vi "extract Z segment with cursors.vi"(6 "sample rate":dbl, 8 "Zmag trajectory":waveform(dbl) caption="元素", 9 "cursor pos":dbl, 10 "data":waveform(dbl)[](array[waveform]), 11 "cursor length":dbl) -> (0 "Z":dbl[](array[numeric]), 4 "Z mag":dbl[](array[numeric]))   [LabVIEW 2017]
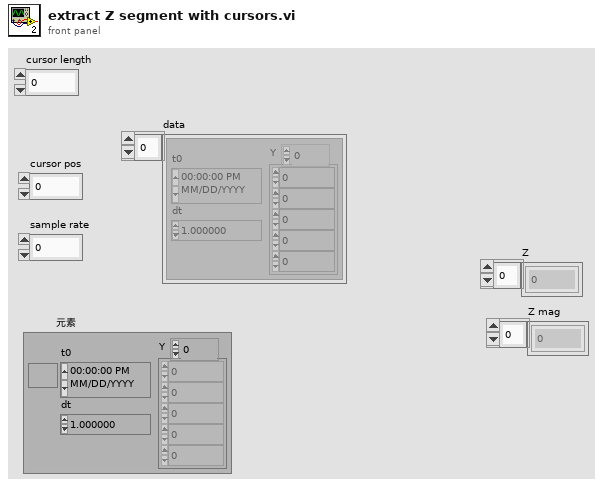
[diagram p1: front panel]
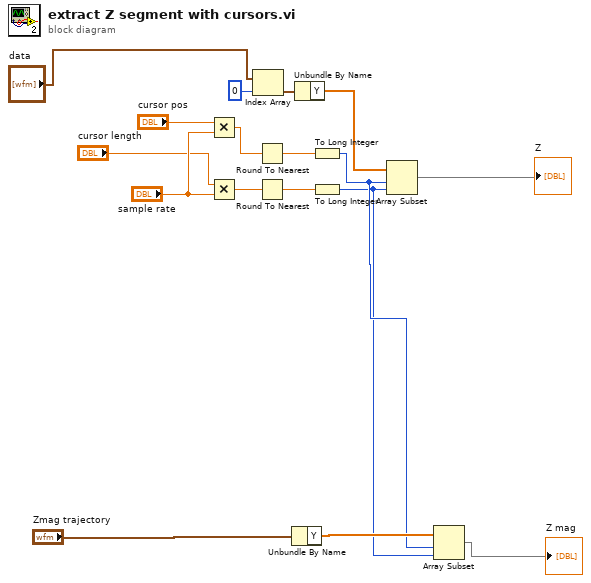
[diagram p0: block diagram]
diagram:
  n1 = Multiply(x="cursor pos", y="sample rate") -> (x*y=w11:dbl)
  n2 = Multiply(x="cursor length", y="sample rate") -> (x*y=w15:dbl)
  n3 = Index Array(array="data", index=0 ("索引")) -> (element=w9:waveform(dbl))
  n4 = Round To Nearest(number=w11) -> (nearest integer value=w12:dbl)
  n5 = Round To Nearest(number=w15) -> (nearest integer value=w14:dbl)
  n6 = Unbundle By Name("Zmag trajectory") -> ("Y"=w5:dbl[])
  n7 = Unbundle By Name(w9) -> ("Y"=w13:dbl[])
  n8 = To Long Integer(number=w12) -> (32bit integer=w4:i32)
  n9 = To Long Integer(number=w14) -> (32bit integer=w3:i32)
  n10 = Array Subset(array=w13, index=w4, length=w3) -> (→"Z":dbl[])
  n11 = Array Subset(array=w5, index=w4, length=w3) -> (→"Z mag":dbl[])
